vi "Compute.vi"(8 "error in (no error)":errorcluster, 9 "Data Channels":T1, 10 "x-var":dbl, 11 "Average in":refnum<class "Average.lvclass">) -> (0 "error out":errorcluster, 1 "Add'l Data Channels":T1, 3 "Average out":refnum<class "Average.lvclass">)   [LabVIEW 2009, in "Average.lvclass"]
doc: "Given a data channel and an x-coordinate, compute and return one or more new data channels."
uses:
  Average.lvclass
  Instruments/Utility Classes/Readable/Data Channels.ctl
  Instruments/Utility Classes/Readable/Data Channel.ctl
  Instruments/Utility Classes/Readable/Data Point.ctl
  Instruments/Utility Classes/Readable/Readable.lvclass
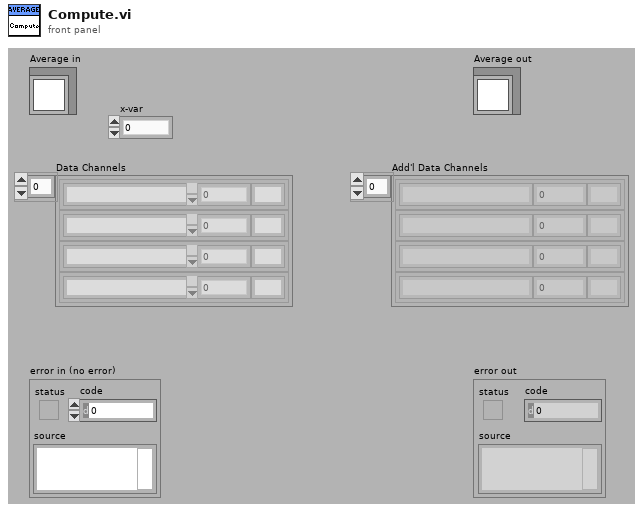
[diagram p1: front panel]
types:
  T1 = typedef "Readable.lvclass/Data Channels.ctl" = T2[]
  T2 = typedef "Readable.lvclass/Data Channel.ctl" = cluster{"Name":string, "Data Point":T3, "Unit":string}
  T3 = typedef "Readable.lvclass/Data Point.ctl" = dbl
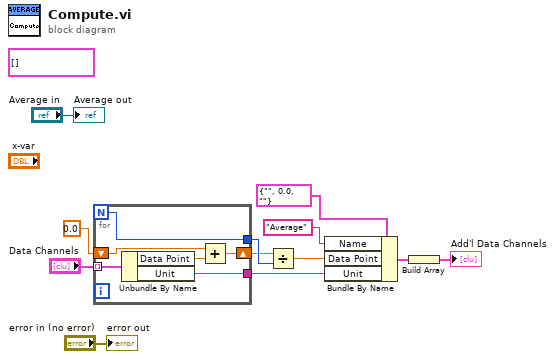
[diagram p0: block diagram]
diagram:
  (unwired) T1 [] ("Data Channels")
  n1 = for {
    N -> [w14]
    tunnel: "Data Channels" -> [w18] mode=indexing
    shift-right: [w16] -> w10
    shift-left: T3 0.0 ("Data Point") -> [w15]
    tunnel: [w14] -> w11
    tunnel: [w13] -> w6
    n2 = Unbundle By Name(w18) -> ("Data Point"=w17:T3, "Unit"=w13:string)
    n3 = Add(x=w15, y=w17) -> (x+y=w16:T3)
  }
  n4 = Divide(x=w10, y=w11) -> (x/y=w5:T3)
  n5 = Bundle By Name(cluster=T2 {"Name"="", "Data Point"=0.0, "Unit"=""} ("Data Channel"), "Name"="Average", "Data Point"=w5, "Unit"=w6) -> (w3:T2)
  n6 = Build Array(w3) -> (→"Add'l Data Channels":T2[])
  "error out" <- "error in (no error)"
  "Average out" <- "Average in"
